vi "Data Receiver.vi"() -> ()   [LabVIEW 2018]
panel:
  out "Received Data":sgl[][](graph)
  out "Data Recieved":sgl[][](graph)
  in  "Stop":bool
  # "Overview: Demonstrates the use of the UDP functions to receive data over a UDP connection.\nInstructions:\n1. Ensure Data Sender.vi is already running.\n2. Run the VI.\n3. Click Stop to stop the VI."
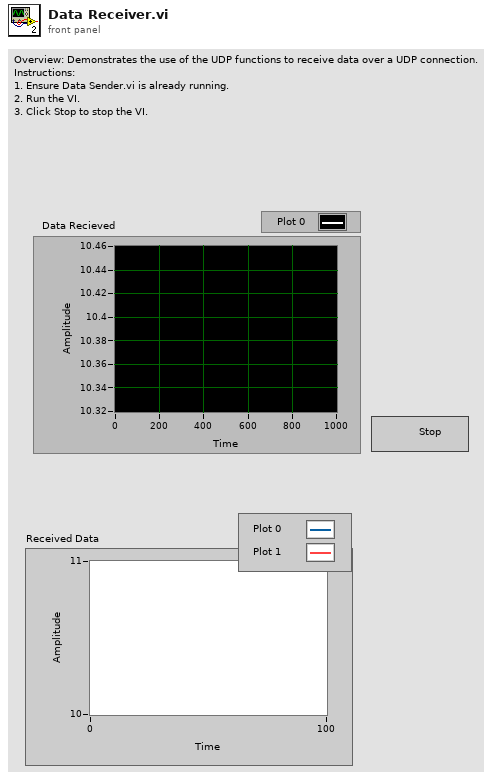
[diagram p1: front panel]
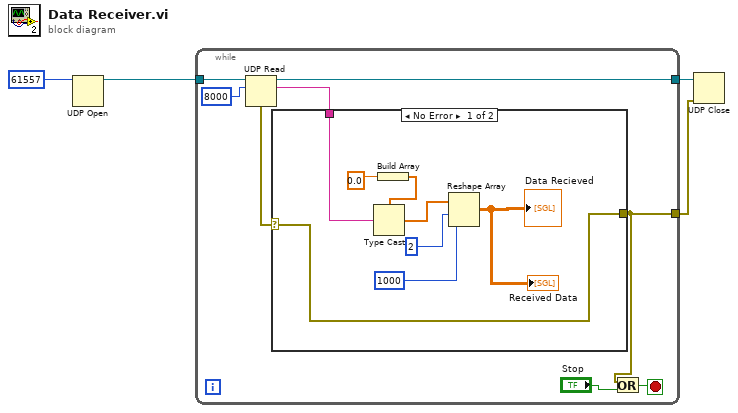
[diagram p0: block diagram]
diagram:
  n1 = UDP Open(11:u16 61557 ("port")) -> (port=w3:refnum<k16>)  [unwired: 4 in, 2 out]
  n2 = while {
    tunnel: w3 -> [w12]
    tunnel: [w11] -> w2
    tunnel: [w7] -> w1
    stop <- w8 stop-if-true
    n3 = UDP Read(connection ID=w12, max size (548)=8000) -> (data out=w10:string, error out=w9:errorcluster, 3:w11:refnum<k16>)  [unwired: 2 in, 2 out]
    n4 = case shown="No Error" w9 {
      selector: w9 -> [w14 w21]
      tunnel: w10 -> [w19 _]
      tunnel: [w14 w21] -> w7
      frame No Error {
        n5 = Build Array(sgl 0.0) -> (w15:sgl[])
        n6 = Type Cast(type=w15, x=w19) -> (*(type *) &x=w17:sgl[])
        n7 = Reshape Array(w17, 2, 1000) -> (→"Data Recieved" →"Received Data":sgl[][])
      }
      frame Error {
      }
    }
    n8 = Or(x=w7, y="Stop") -> (x .or. y?=w8:bool)
  }
  n9 = UDP Close(connection ID=w2, 8:w1) -> ()  [unwired: 2 out]
